vi "Read StateStateRef.vi"(8 "error in (no error)":errorcluster, 11 "Receiver in":refnum<class "Receiver.lvclass">) -> (0 "error out":errorcluster, 2 "StateStateRef":refnum<vi>, 3 "Receiver out":refnum<class "Receiver.lvclass">)   [LabVIEW 2013]
uses:
  Receiver.lvclass
  ReceiverState/StateState.ctl
  Connect Command/Connect Command.lvclass
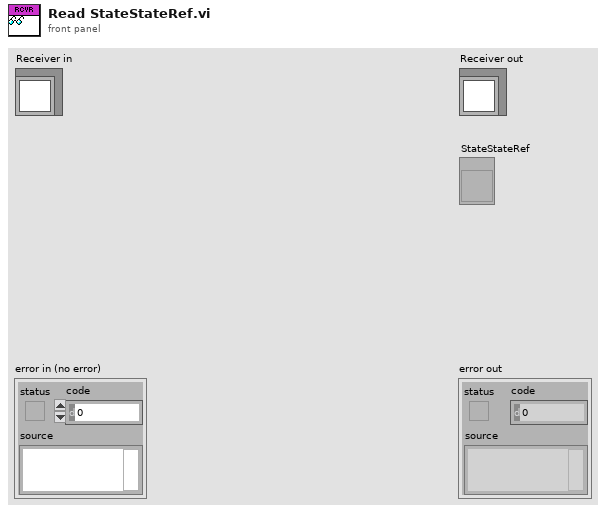
[diagram p1: front panel]
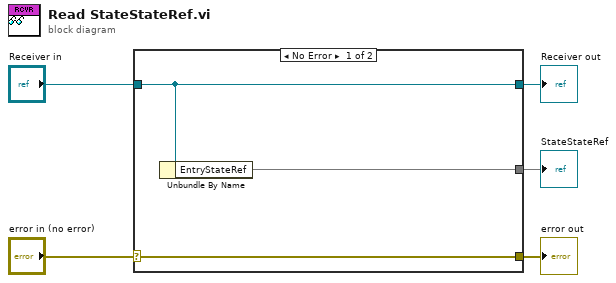
[diagram p0: block diagram]
diagram:
  n1 = case shown="No Error" "error in (no error)" {
    selector: "error in (no error)" -> [w8 w9]
    tunnel: [w8 w9] -> w4
    tunnel: [w7 w10] -> w2
    tunnel: "Receiver in" -> [w7 w10]
    tunnel: [w6 _] -> w1
    frame No Error {
      n2 = Unbundle By Name(w7) -> ("EntryStateRef"=w6)
    }
    frame Error {
    }
  }
  "error out" <- w4
  "Receiver out" <- w2
  "StateStateRef" <- w1
